vi "non_FPGA_VI_v2.vi"() -> ()   [LabVIEW 2020]
uses:
  c5c29772-c0b0-45e0-ac49-cc5077cfdad3.vi
  <vilib>/Array/Sort 2D Array - Pop Stack.vi
  <vilib>/Array/Sort 2D Array - Push Stack.vi
  c5c29772-c0b0-45e0-ac49-cc5077cfdad3.vi/269d4b3b-47f5-49e3-8884-44851e4dd9d5.vi
  c5c29772-c0b0-45e0-ac49-cc5077cfdad3.vi/6d99389c-673d-4efb-bf33-19b32bcf4cf8.vi
  <vilib>/Analysis/NI_AALBase.lvlib
panel:
  out "sorted array":dbl[](graph)
  out "sorted array index":i32[](array[numeric])
  out "sorted array img":fxp<+/-,32,21>[](array[numeric])
  out "sorted array real":fxp<+/-,32,21>[](array[numeric])
  out "sorted 2D array":dbl[][](array[numeric])
  out "appended array":dbl[][](array[numeric])
  out "Array 3":i32[](array[numeric])
  out "sorted array":dbl[](array[numeric])
  out "Array":dbl[](array[numeric])
  out "uniform white noise":dbl[](array[numeric])
  out "array input":dbl[](graph)
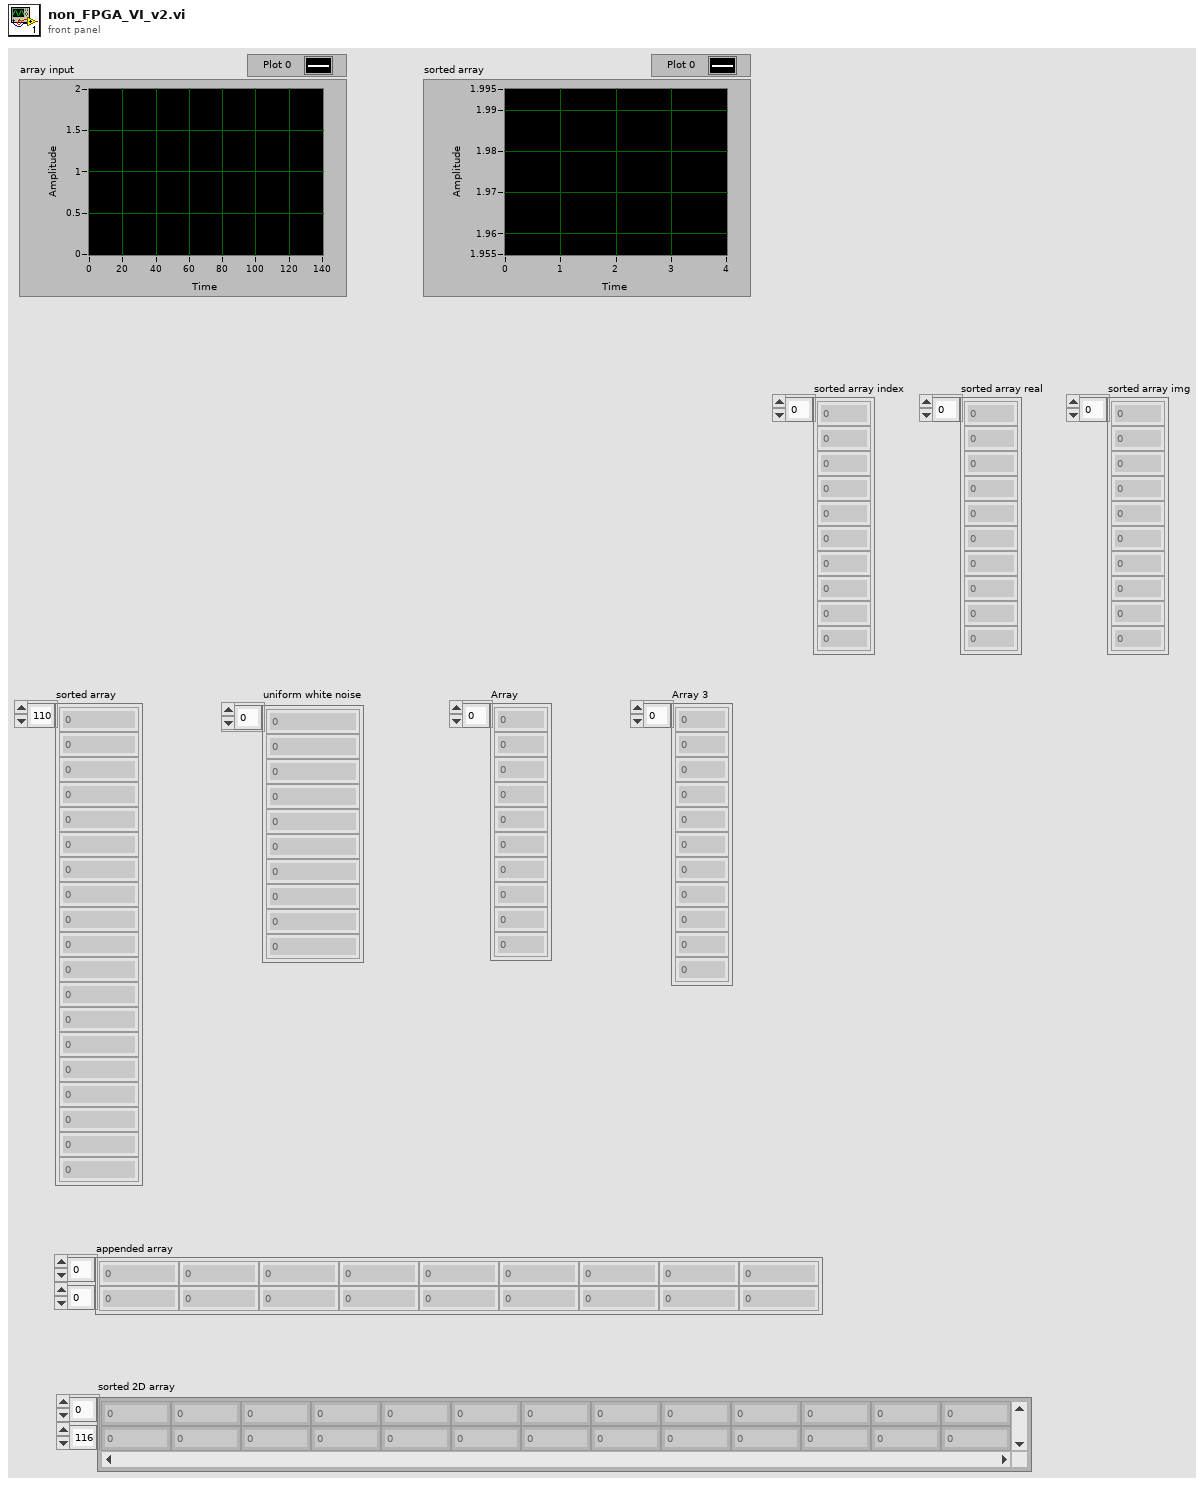
[diagram p1: front panel]
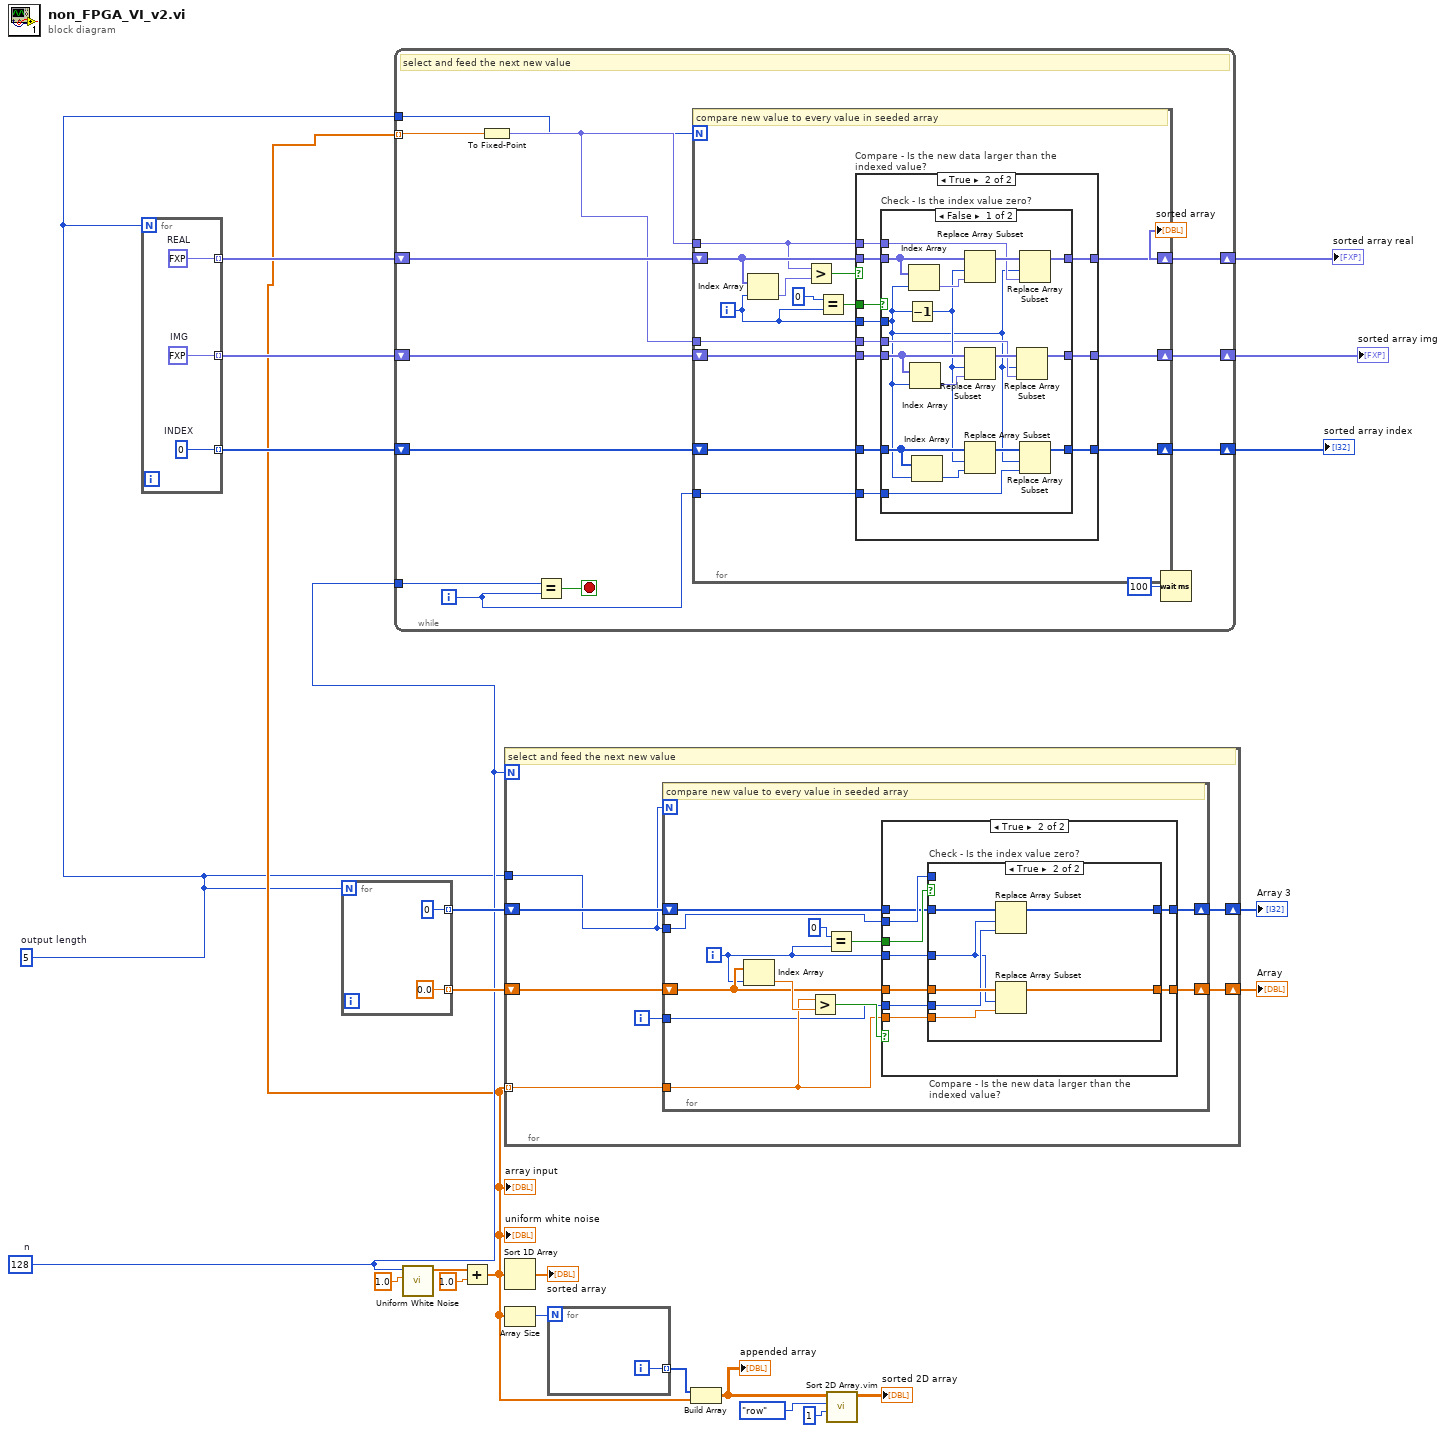
[diagram p0: block diagram]
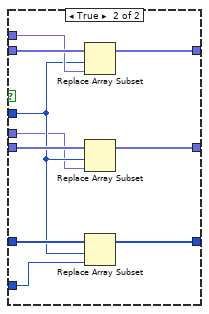
[diagram p3: hidden frame]
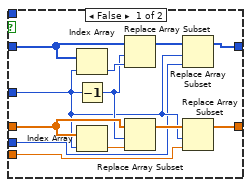
[diagram p5: hidden frame]
diagram:
  w2 = 5  # output length
  w4 = 128  # n
  n1 = for {
    N: w2 -> [_]
    tunnel: [w26] -> w8 mode=indexing
    tunnel: [w25] -> w9 mode=indexing
    tunnel: [w24] -> w7 mode=indexing
    w24 = fxp<+/-,32,21> 0.0  # IMG
    w25 = 0  # INDEX
    w26 = fxp<+/-,32,21> 0.0  # REAL
  }
  n2 = for {
    N: w2 -> [_]
    tunnel: [0.0 ("amplitude")] -> w22 mode=indexing
    tunnel: [0] -> w17 mode=indexing
  }
  n3 = call <vilib>:"Uniform White Noise.vi"("amplitude"=1.0, "samples"=w4) -> ("uniform white noise"=w15:dbl[])  [unwired: 8 in, 1 out]
  n4 = Add(x=w15, y=1.0 ("amplitude")) -> (x+y=w3:dbl[])
  "array input" <- w3
  "uniform white noise" <- w3
  n5 = while {
    shift-right: [w30] -> w1
    shift-left: w8 -> [w41]
    shift-right: [w40] -> w6
    shift-left: w9 -> [w39]
    tunnel: w4 -> [w37]
    shift-right: [w35] -> w5
    shift-left: w7 -> [w34]
    tunnel: w3 -> [w33] mode=indexing
    tunnel: w2 -> [w31]
    i -> [w38]
    stop <- w36 stop-if-true
    # "select and feed the next new value"
    n6 = To Fixed-Point(number=w33) -> (fixed-point=w32:fxp<+/-,32,16>)  [unwired: 1 in]
    n7 = Equal?(x=w37, y=w38) -> (x = y?=w36:bool)
    n8 = for {
      N: w31 -> [_]
      tunnel: w32 -> [w52]
      shift-right: [w51] -> w30
      shift-left: w41 -> [w53]
      tunnel: w38 -> [w49]
      shift-right: [w47] -> w40
      shift-left: w39 -> [w48]
      shift-right: [w44] -> w35
      shift-left: w34 -> [w43]
      tunnel: w32 -> [w42]
      i -> [w50]
      # "compare new value to every value in seeded array"
      n9 = Index Array(array=w53, index=w50) -> (element=w55:fxp<+/-,32,21>)
      n10 = Greater?(x=w52, y=w55) -> (0:w54:bool)
      n11 = Equal?(x=0, y=w50) -> (x = y?=w45:bool)
      n12 = case "Compare - Is the new data larger than the indexed value?" shown="True" w54 {
        tunnel: w53 -> [w58 w68]
        tunnel: w45 -> [_ w69]
        tunnel: w52 -> [_ w67]
        tunnel: w50 -> [_ w66]
        tunnel: [w58 w65] -> w51
        tunnel: w49 -> [_ w64]
        tunnel: w48 -> [w57 w63]
        tunnel: [w57 w62] -> w47
        tunnel: [w56 w61] -> w44
        tunnel: w43 -> [w56 w60]
        tunnel: w42 -> [_ w59]
        frame False {
        }
        frame True {
          n13 = case "Check - Is the index value zero?" shown="False" w69 {
            tunnel: w68 -> [w86 w96]
            tunnel: w67 -> [w83 w95]
            tunnel: w66 -> [w70 w89]
            tunnel: [w82 w94] -> w65
            tunnel: w64 -> [w77 w93]
            tunnel: w63 -> [w79 w92]
            tunnel: [w78 w91] -> w62
            tunnel: [w72 w87] -> w61
            tunnel: w60 -> [w76 w90]
            tunnel: w59 -> [w71 w88]
            frame False {
              n14 = Decrement(x=w70) -> (x-1=w74:i32)
              n15 = Index Array(array=w86, index=w70) -> (element=w85:fxp<+/-,32,21>)
              n16 = Index Array(array=w76, index=w70) -> (element=w75:fxp<+/-,32,21>)
              n17 = Index Array(array=w79, index=w70) -> (element=w81:i32)
              n18 = Replace Array Subset(array=w86, new element=w85, index=w74) -> (w84:fxp<+/-,32,21>[])
              n19 = Replace Array Subset(array=w76, new element=w75, index=w74) -> (w73:fxp<+/-,32,21>[])
              n20 = Replace Array Subset(array=w79, new element=w81, index=w74) -> (w80:i32[])
              n21 = Replace Array Subset(array=w73, new element=w71, index=w70) -> (w72:fxp<+/-,32,21>[])
              n22 = Replace Array Subset(array=w84, new element=w83, index=w70) -> (w82:fxp<+/-,32,21>[])
              n23 = Replace Array Subset(array=w80, new element=w77, index=w70) -> (w78:i32[])
            }
            frame True {
              n24 = Replace Array Subset(array=w96, new element=w95, index=w89) -> (w94:fxp<+/-,32,21>[])
              n25 = Replace Array Subset(array=w90, new element=w88, index=w89) -> (w87:fxp<+/-,32,21>[])
              n26 = Replace Array Subset(array=w92, new element=w93, index=w89) -> (w91:i32[])
            }
          }
        }
      }
    }
    "sorted array" <- w30
    n27 = Wait (ms)(milliseconds to wait=u32 100) -> ()  [unwired: 1 out]
  }
  "sorted array real" <- w1
  "sorted array img" <- w5
  "sorted array index" <- w6
  n28 = for {
    N: w4 -> [_]
    tunnel: w3 -> [w103] mode=indexing
    shift-right: [w101] -> w21
    shift-left: w22 -> [w102]
    shift-right: [w99] -> w18
    shift-left: w17 -> [w98]
    tunnel: w2 -> [w97]
    i -> [w100]
    # "select and feed the next new value"
    n29 = for {
      N: w97 -> [_]
      tunnel: w103 -> [w110]
      tunnel: w97 -> [w108]
      shift-right: [w109] -> w101
      shift-left: w102 -> [w113]
      tunnel: w100 -> [w106]
      shift-right: [w104] -> w99
      shift-left: w98 -> [w105]
      i -> [w107]
      # "compare new value to every value in seeded array"
      n30 = Index Array(array=w113, index=w107) -> (element=w115:dbl)
      n31 = Greater?(x=w110, y=w115) -> (0:w114:bool)
      n32 = Equal?(x=0, y=w107) -> (x = y?=w111:bool)
      n33 = case "Compare - Is the new data larger than the indexed value?" shown="True" w114 {
        tunnel: w113 -> [w117 w125]
        tunnel: w111 -> [_ w126]
        tunnel: w108 -> [_ w124]
        tunnel: w110 -> [_ w123]
        tunnel: w107 -> [_ w122]
        tunnel: [w117 w121] -> w109
        tunnel: w106 -> [_ w120]
        tunnel: w105 -> [w116 w119]
        tunnel: [w116 w118] -> w104
        frame False {
        }
        frame True {
          n34 = case "Check - Is the index value zero?" shown="True" w126 {
            tunnel: w125 -> [w138 w145]
            tunnel: w124 -> [_ _]
            tunnel: w123 -> [w135 w144]
            tunnel: w122 -> [w128 w141]
            tunnel: [w134 w143] -> w121
            tunnel: w120 -> [w127 w142]
            tunnel: w119 -> [w131 w140]
            tunnel: [w130 w139] -> w118
            frame False {
              n35 = Index Array(array=w131, index=w128) -> (element=w133:i32)
              n36 = Decrement(x=w128) -> (x-1=w129:i32)
              n37 = Index Array(array=w138, index=w128) -> (element=w137:dbl)
              n38 = Replace Array Subset(array=w131, new element=w133, index=w129) -> (w132:i32[])
              n39 = Replace Array Subset(array=w138, new element=w137, index=w129) -> (w136:dbl[])
              n40 = Replace Array Subset(array=w132, new element=w127, index=w128) -> (w130:i32[])
              n41 = Replace Array Subset(array=w136, new element=w135, index=w128) -> (w134:dbl[])
            }
            frame True {
              n42 = Replace Array Subset(array=w140, new element=w142, index=w141) -> (w139:i32[])
              n43 = Replace Array Subset(array=w145, new element=w144, index=w141) -> (w143:dbl[])
            }
          }
        }
      }
    }
  }
  "Array" <- w21
  "Array 3" <- w18
  n44 = Sort 1D Array(array=w3) -> (sorted array=→"sorted array":dbl[])
  n45 = Array Size(array=w3) -> (size(s)=w16:i32)
  n46 = for {
    N: w16 -> [_]
    tunnel: [w146] -> w14 mode=indexing
    i -> [w146]
  }
  n47 = Build Array(w14, w3) -> (w13:dbl[][])
  "appended array" <- w13
  n48 = call "Sort 2D Array.vim"("index"=1, "dimension to index (column)"=enum16{"column", "row"}."row", "2D array"=w13) -> ("sorted 2D array"=→"sorted 2D array":dbl[][])  [unwired: 7 in, 1 out]
